vi "Handle Command.vi"(8 "error in":errorcluster, 10 "CMD in":refnum<class "Change Samples per Cycle CMD.lvclass">, 11 "Object In":refnum<class>) -> (0 "error out":errorcluster, 1 "Command Successful?":bool, 2 "CMD out":refnum<class "Change Samples per Cycle CMD.lvclass">, 3 "Object Out":refnum<class>)   [LabVIEW 2017, in "gCRDS.lvlib" / "Change Samples per Cycle CMD.lvclass"]
doc: "This VI will contain the code used to actually execute the request. If the request is successful, this will be indicated by the boolean output <b>Command Successful?</b>. The boolean output can then be used by the <b>Command Reply</b> which sends a reply if the reply queue is valid."
uses:
  Change Samples per Cycle CMD.lvclass
  gCRD.lvclass
  C:/Program Files (x86)/National Instruments/LabVIEW 2017/vi.lib/MSR Consulting, LLC/General Reuse/Instrument/Instrument.lvclass
  <vilib>/MSR Consulting, LLC/General Reuse/Instrument/Instrument.lvclass/Instrument.ctl
  gCRD.lvclass/gCRD.ctl
  Change Samples per Cycle CMD.lvclass/Change Samples per Cycle CMD.ctl
  Accessors/Write SamplesPerCycle.vi
  <vilib>/MSR Consulting, LLC/General Reuse/Instrument/Read ExtCom.vi
  <vilib>/MSR Consulting, LLC/General Reuse/Instrument/Read Log Session.vi
  Accessors/Read RepRate.vi
  <vilib>/MSR Consulting, LLC/General Reuse/Session APIs/_Session Fwk/Session - Root.lvclass
  <vilib>/MSR Consulting, LLC/General Reuse/Session APIs/Session Log/System Log.lvclass
  Change Rep Rate/Change Laser Rep Rate CMD.lvclass
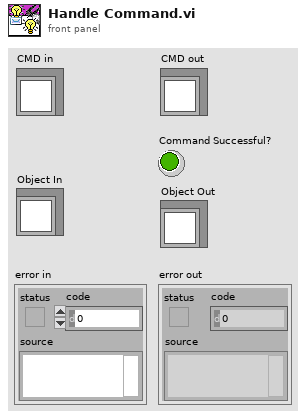
[diagram p1: front panel]
types:
  T1 = typedef "Session - Root.lvclass/Session Handle.ctl" = refnum<data-value>
  T2 = cluster{"tag":string, "section":string, "data":variant}
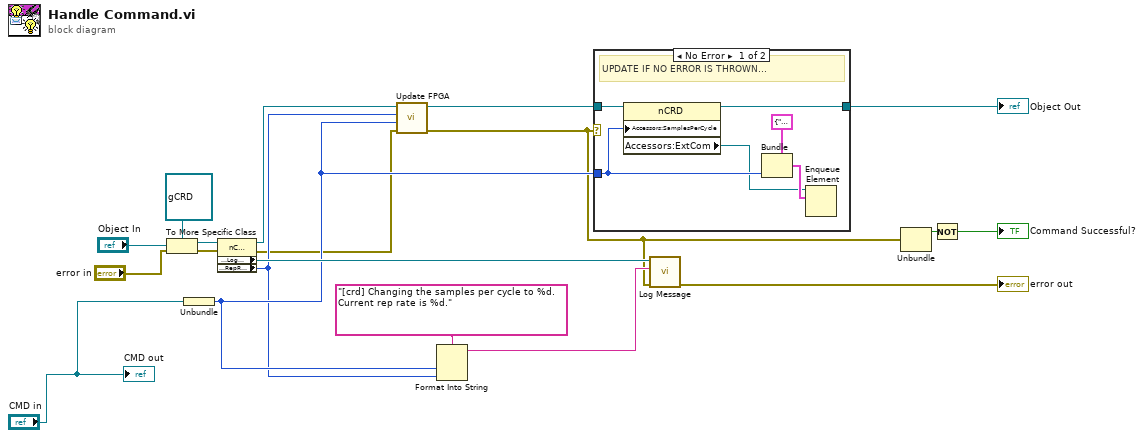
[diagram p0: block diagram]
diagram:
  n1 = To More Specific Class(target class=refnum<class "gCRD.lvclass"> refnum ("gCRDS.lvlib:nCRD"), reference="Object In", error in="error in") -> (specific class reference=w19:refnum<class "gCRD.lvclass">, error out=w18:errorcluster)
  n2 = Unbundle("CMD in") -> (w4:u16)
  n3 = property class="nCRD"(reference=w19, error in=w18) -> (reference out=w6:refnum<class "gCRD.lvclass">, error out=w2:errorcluster, "Accessors:Log Session"=w17:T1, "Accessors:RepRate"=w3:u16)
  n4 = call "Update FPGA.vi"("error in"=w2, "Samples per Cycle"=w4, "RepRate"=w3, "gCRDS"=w6) -> ("error out"=w1:errorcluster, "gCRDS"=w5:refnum<class "gCRD.lvclass">)  [unwired: 6 in]
  n5 = Format Into String(format string="[crd] Changing the samples per cycle to %d.  Current rep rate is %d.", w4, w3) -> (resulting string=w15:string)  [unwired: 2 in, 1 out]
  n6 = case shown="No Error" w1 {
    tunnel: w5 -> [w23 w26]
    tunnel: [w22 w26] -> w9
    tunnel: w4 -> [w21 _]
    frame No Error {
      # "UPDATE IF NO ERROR IS THROWN..."
      n7 = property class="nCRD"(reference=w23, "Accessors:SamplesPerCycle"=w21) -> (reference out=w22:refnum<class "gCRD.lvclass">, "Accessors:ExtCom"=w20:refnum<queue>)  [unwired: 1 in, 1 out]
      n8 = Bundle(cluster=T2 {"tag"="samp_per_cycle", "section"="crd", "data"=variant} ("element"), "data"=w21) -> (w24:T2)  [unwired: 2 in]
      n9 = Enqueue Element(queue=w20, element=w24) -> ()  [unwired: 2 in, 3 out]
    }
    frame Error {
    }
  }
  "Object Out" <- w9
  n10 = call <vilib>:"Log Message.vi"("error in"=w1, "MSG In"=w15, "session in"=w17) -> ("error out"=→"error out":errorcluster)  [unwired: 7 in, 1 out]
  n11 = Unbundle(w1) -> ("status"=w13:bool)  [unwired: 2 out]
  n12 = Not(x=w13) -> (.not. x?=→"Command Successful?":bool)
  "CMD out" <- "CMD in"
